vi "solar_voy Register (Import).vi"(6 "Suppress Errors? (T)":bool=TRUE, 8 "error in (no error)":errorcluster, 9 "COSMOS_Root (\"\"=Use Default)":path, 10 "Target Name":string, 11 "Voyager Refnum in":T1) -> (0 "error out":errorcluster, 3 "Voyager Refnum out":T1)   [LabVIEW 2018]
doc: "This imports a COSMOS Target's command and telemetry definition files."
uses:
  solar_voy_def/solar_voy_def_ctl PATH.ctl
  solar_voy_ctl Voyager Refnum.ctl
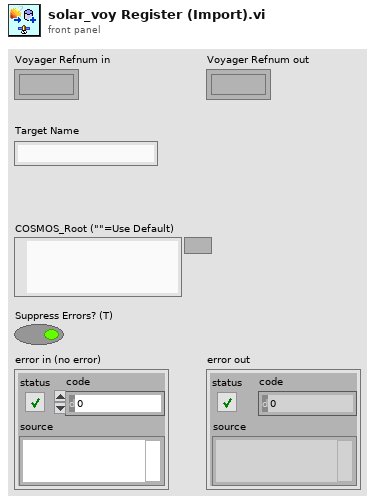
[diagram p1: front panel]
types:
  T1 = typedef "solar_voy_ctl Voyager Refnum.ctl" = refnum<k1>
  T2 = typedef "solar_voy_def_ctl PATH.ctl" = enum8{"..", "config", "config/data", "config/system", "config/targets", "config/targets/TARGET", "config/targets/TARGET/cmd_tlm", "config/targets/TARGET/lib", "config/targets/TARGET/screens", "config/tools", "config/tools/cmd_tlm_server", "config/tools/data_viewer", "config/tools/handbook_creator", "config/tools/launcher", "config/tools/limits_monitor", "config/tools/opengl_builder", "config/tools/script_runner", "config/tools/table_manager", "config/tools/test_runner", "config/tools/tlm_extractor", "config/tools/tlm_grapher", "config/tools/tlm_viewer", "lib", "outputs", "outputs/handbooks", "outputs/logs", "outputs/saved_config", "outputs/tables", "outputs/tmp", "procedures", "tools", "Launcher.bat", "config/system/system.txt", "config/targets/TARGET/cmd_tlm/TARGET_cmd.txt", "config/targets/TARGET/cmd_tlm/TARGET_tlm.txt", "config/targets/TARGET/cmd_tlm_server.txt", "config/targets/TARGET/target.txt", "config/tools/cmd_tlm_server/cmd_tlm_server.txt", "config/tools/data_viewer/data_viewer.txt", "config/tools/handbook_creator/handbook_creator.txt", "config/tools/launcher/launcher.txt", "config/tools/limits_monitor/limits_monitor.txt", "config/tools/opengl_builder/opengl_builder.txt", "config/tools/script_runner/script_runner.txt", "config/tools/table_manager/table_manager.txt", "config/tools/test_runner/test_runner.txt", "config/tools/tlm_extractor/tlm_extractor.txt", "config/tools/tlm_grapher/tlm_grapher.txt", "config/tools/tlm_viewer/tlm_viewer.txt"}
  T3 = typedef "solar_voy_ctl Voyager.ctl" = cluster{"PACKETS":T4[], "COSMOS_Root":path, "CMD_HDR":T9, "TLM_HDR":T9, "TCPs":T10[], "VoyagerIDOffset":cluster{"VoyagerIDOffset":u16[], "Target Names":string[]}}
  T4 = typedef "solar_voy_def_ctl PACKET.ctl" = cluster{"PACKET_ID":T5, "ENDIAN":enum8{"BIG", "LITTLE"}, "DESC":string, "HZRD":bool, "ITEMS":T6[], "NoExport":bool, "last_time":timestamp, "last_count":u32, "last_data":string}
  T5 = typedef "solar_voy_def_ctl PACKET_ID.ctl" = cluster{"ID":u16, "CMD":enum8{"CMD", "TLM"}, "TARGET":string, "PACKET":string}
  T6 = typedef "solar_voy_def_ctl ITEM.ctl" = cluster{"NAME":string, "OFFSET":i32, "SIZE":i32, "TYPE":T7, "EACH_SIZE":i32, "LVTYPE":T8, "MIN":dbl, "MAX":dbl, "DEFAULT":string, "DESC":string, "ID":bool, "MODIFIERS":variant, "last_value":variant}
  T7 = typedef "solar_voy_def_ctl ITEM TYPE.ctl" = enum8{"BLOCK", "INT", "UINT", "FLOAT", "STRING"}
  T8 = typedef "solar_type Item Type.ctl" = enum16{"NULL", "UNKNOWN", "CLUSTER", "I8", "I16", "I32", "I64", "U8", "U16", "U32", "U64", "U8_ENUM", "U16_ENUM", "U32_ENUM", "SGL", "DBL", "BOOLEAN", "STRING", "PATH", "VISA", "TAG", "TIME", "I8_1D", "I16_1D", "I32_1D", "I64_1D", "U8_1D", "U16_1D", "U32_1D", "U64_1D", "U8_ENUM_1D", "U16_ENUM_1D", "U32_ENUM_1D", "SGL_1D", "DBL_1D", "BOOLEAN_1D", "STRING_1D", "PATH_1D", "VISA_1D", "TAG_1D", "TIME_1D", "I8_2D", "I16_2D", "I32_2D", "I64_2D", "U8_2D", "U16_2D", "U32_2D", "U64_2D", "U8_ENUM_2D", "U16_ENUM_2D", "U32_ENUM_2D", "SGL_2D", "DBL_2D", "BOOLEAN_2D", "STRING_2D", "PATH_2D", "VISA_2D", "TAG_2D", "TIME_2D"}
  T9 = typedef "solar_voy_def_ctl HDR.ctl" = cluster{"ITEMS":T6[], "LENGTH_NAME":string, "LENGTH_VALUE_OFFSET":i32, "ID_NAME":string, "ENDIAN":enum8{"BIG", "LITTLE"}, "GUID_NAME":string, "DEFAULT_TARGET":string, "DEFAULT_PACKET":string, "DEFAULT_ERROR":string}
  T10 = typedef "solar_voy_ctl TCP.ctl" = cluster{"Connected":bool, "Port":u16, "Listener":refnum<k5>, "ServerIP":string, "TCP":refnum<k5>, "Setup":T11, "VIRefnum":refnum<vi>, "TARGETS_CMD":string[], "TARGETS_TLM":string[]}
  T11 = typedef "solar_voy_ctl Port Setup.ctl" = enum8{"SERVER", "CLIENT", "SERVER_CMD", "SERVER_TLM"}
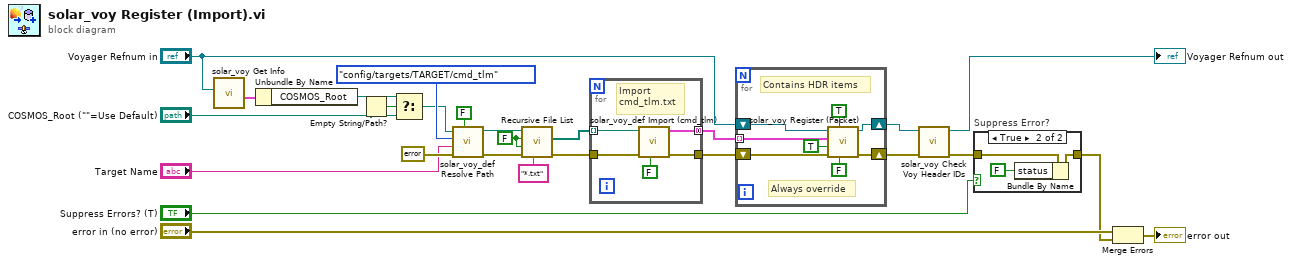
[diagram p0: block diagram]
diagram:
  w8 = FALSE ("Treat LLBs as Folders?")
  n1 = call "solar_voy Get Info.vi"("Voyager Refnum"="Voyager Refnum in") -> ("Voyager"=w22:T3)  [unwired: 8 in, 2 out]
  n2 = Unbundle By Name(w22) -> ("COSMOS_Root"=w14:path)
  n3 = Empty String/Path?(string/path="COSMOS_Root (\"\"=Use Default)") -> (empty?=w16:bool)
  n4 = Select(t=w14, s=w16, f="COSMOS_Root (\"\"=Use Default)") -> (s? t:f=w13:path)
  n5 = call "solar_voy_def Resolve Path.vi"("Create Folder? (T)"=FALSE, "error in (no error)"=errorcluster {"status"=FALSE, "code"=0, "source"=""} ("error out"), "TARGET"="Target Name", "PATH (..=Root)"=solar_voy_def_ctl_PATH."config/targets/TARGET/cmd_tlm", "COSMOS_ROOT"=w13) -> ("error out"=w11:errorcluster, "Resolved Path"=w10:path)  [unwired: 5 in]
  n6 = call <vilib>:"Recursive File List.vi"("pattern"="*.txt", "error in (no error)"=w11, "Continue Recursing on Error? (F)"=w8, "Treat LLBs as Folders?"=w8, "Folder Path"=w10) -> ("error out"=w7:errorcluster, "All Files in Dir"=w6:path[])  [unwired: 2 in, 3 out]
  n7 = for {
    tunnel: [w31] -> w18
    tunnel: [w30] -> w17 mode=concatenating
    tunnel: w7 -> [w28]
    tunnel: w6 -> [w27] mode=indexing
    # "Import\ncmd_tlm.txt"
    n8 = call "solar_voy_def Import (cmd_tlm).vi"("Suppress Errors? (T)"=FALSE, "error in (no error)"=w28, "cmd_tlm.txt"=w27) -> ("error out"=w31:errorcluster, "PACKETS"=w30:T4[])  [unwired: 7 in]
  }
  n9 = for {
    shift-right: [w38] -> w4
    shift-left: w18 -> [w39]
    tunnel: w17 -> [w36] mode=indexing
    shift-right: [w33] -> w2
    shift-left: "Voyager Refnum in" -> [w34]
    # "Contains HDR items"
    # "Always override"
    n10 = call "solar_voy Register (Packet).vi"("Suppress Errors? (T)"=FALSE, "Contains HDR? (F)"=TRUE, "error in (no error)"=w39, "Override If Exists? (F)"=TRUE, "PACKET (No HDR)"=w36, "Voyager Refnum in"=w34) -> ("error out"=w38:errorcluster, "Voyager Refnum out"=w33:T1)  [unwired: 4 in]
  }
  n11 = call "solar_voy Check Voy Header IDs.vi"("error in"=w4, "Voyager Refnum"=w2) -> ("Error out"=w3:errorcluster, "Voyager Refnum out"=→"Voyager Refnum out":T1)  [unwired: 8 in]
  n12 = case "Suppress Error?" shown="True" "Suppress Errors? (T)" {
    tunnel: w3 -> [w40 w43]
    tunnel: [w40 w42] -> w24
    frame False {
    }
    frame True {
      n13 = Bundle By Name(cluster=w43, "status"=FALSE) -> (w42:errorcluster)
    }
  }
  n14 = Merge Errors("error in (no error)", w24) -> (→"error out":errorcluster)
